vi "Pockels_test.vi"() -> ()   [LabVIEW 2011]
uses:
  <vilib>/DAQmx/write.llb/DAQmx Write (Digital Bool 1Line 1Point).vi
  <vilib>/DAQmx/write.llb/DAQmx Write (Analog DBL 1Chan 1Samp).vi
  <vilib>/DAQmx/create/channels.llb/DAQmx Create Channel (AO-Voltage-Basic).vi
  <vilib>/DAQmx/create/channels.llb/DAQmx Create Channel (DO-Digital Output).vi
  <vilib>/DAQmx/miscellaneous.llb/DAQmx Fill In Error Info.vi
panel:
  in  "Shutter":bool
  in  "Shutter digital line":tag="PXI-6229/port0/line0"
  in  "Quit":bool
  in  "PockelsVolt":dbl(slide) min=0.0 max=1.0 step=0.005 scale=0.0..1.0
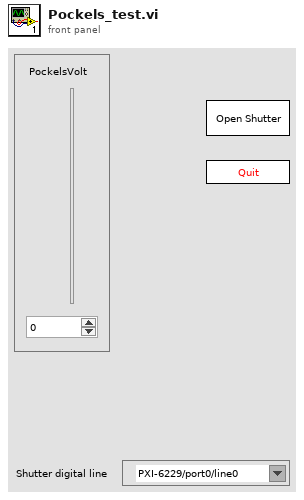
[diagram p1: front panel]
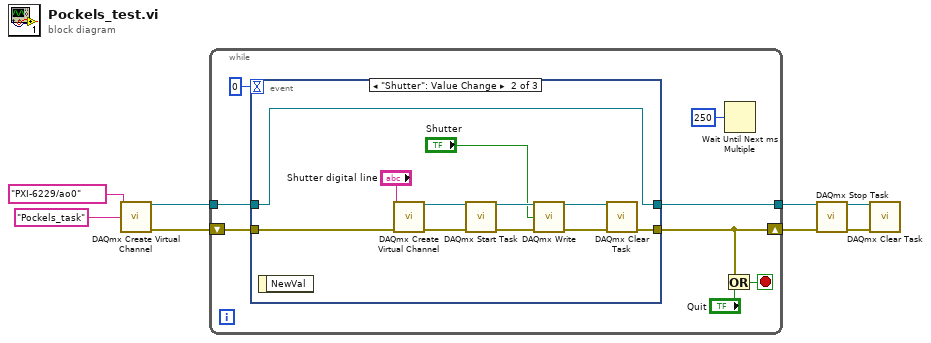
[diagram p0: block diagram]
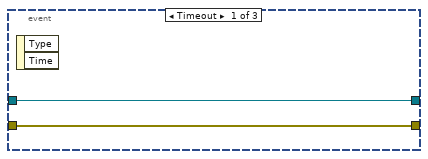
[diagram p2: hidden frame]
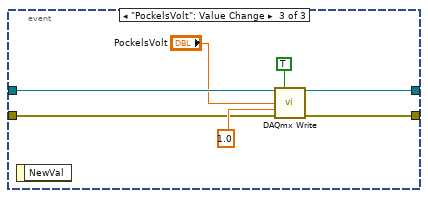
[diagram p3: hidden frame]
diagram:
  n1 = call-poly <vilib>:"DAQmx Create Virtual Channel.vi"("physical channels"=tag "PXI-6229/ao0", "name to assign"="Pockels_task") -> ("task out"=w5:refnum<k21>, "error out"=w6:errorcluster)  [unwired: 12 in]
  n2 = while {
    shift-right: [w11] -> w4
    shift-left: w6 -> [w16]
    tunnel: w5 -> [w15]
    tunnel: [w14] -> w3
    stop <- w9 stop-if-true
    n3 = event shown="[1] \"Shutter\": Value Change" {
      selector: _ -> [_ _ _]
      dyn-events: _ -> [_ _ _]
      timeout: 0 -> [_ _ _]
      tunnel: w16 -> [w17 w22 w34]
      tunnel: w15 -> [w18 w19 w33]
      tunnel: [w18 w19 w31] -> w14
      tunnel: [w17 w20 w30] -> w11
      event Timeout {
        n4 = event-data() -> ()  [unwired: 1 in, 2 out]
      }
      event "Shutter": Value Change {
        n5 = event-data() -> ()  [unwired: 1 in, 1 out]
        n6 = call-poly <vilib>:"DAQmx Create Virtual Channel.vi"("lines"="Shutter digital line", "error in"=w22) -> ("task out"=w23:refnum<k21>, "error out"=w24:errorcluster)  [unwired: 12 in]
        n7 = call <vilib>:"DAQmx Start Task.vi"("task/channels in"=w23, "error in"=w24) -> ("task out"=w25:refnum<k21>, "error out"=w26:errorcluster)  [unwired: 12 in]
        n8 = call-poly <vilib>:"DAQmx Write.vi"("task/channels in"=w25, "data"="Shutter", "error in"=w26) -> ("task out"=w27:refnum<k21>, "error out"=w28:errorcluster)  [unwired: 10 in, 1 out]
        n9 = call <vilib>:"DAQmx Clear Task.vi"("task in"=w27, "error in"=w28) -> ("error out"=w20:errorcluster)  [unwired: 13 in]
      }
      event "PockelsVolt": Value Change {
        n10 = event-data() -> ()  [unwired: 1 in, 1 out]
        n11 = call-poly <vilib>:"DAQmx Write.vi"("task/channels in"=w33, "auto start"=TRUE, "data"="PockelsVolt", "timeout"=1.0, "error in"=w34) -> ("task out"=w31:refnum<k21>, "error out"=w30:errorcluster)  [unwired: 8 in, 1 out]
      }
    }
    n12 = Or(x=w11, y="Quit") -> (x .or. y?=w9:bool)
    n13 = Wait Until Next ms Multiple(millisecond multiple=u32 250) -> ()  [unwired: 1 out]
  }
  n14 = call <vilib>:"DAQmx Stop Task.vi"("task/channels in"=w3, "error in"=w4) -> ("task out"=w1:refnum<k21>, "error out"=w2:errorcluster)  [unwired: 12 in]
  n15 = call <vilib>:"DAQmx Clear Task.vi"("task in"=w1, "error in"=w2) -> ()  [unwired: 13 in, 1 out]
